vi "FGV_MCA.vi"(8 "Error In":errorcluster, 9 "TAC Settings":cluster{"Full Scale (ns)":dbl, "# bins":i32}={"Full Scale (ns)"=1000.0, "# bins"=1000} {"# bins" min=1 max=65535 step=1; "Full Scale (ns)" format="%0.2f"}, 10 "MCA Action":T1) -> (0 "error out":errorcluster, 1 "Delta Time (s)":dbl, 2 "Total Time (s)":dbl, 3 "Coincidence Signal":cluster{"Axis":dbl[], i32[]}(graph), 5 "Paused":bool)   [LabVIEW 2014]
doc: "Functional Global Variable or Action Engine implementation of a Multi-Channel Analyser that uses a DAQcard's analog input triggered by a logic pulse received on digital trigger input.\n\nBy default the analog input range is set from 0 V to 10 V full scale. The read trigger digital pulse arrives on PFI14 (pin 41), and the analog differential read on AI0+ and AI0-.\n\nTested on both M and X series DAQcards."
uses:
  Typedef_MCAControl.ctl
  <vilib>/DAQmx/read.llb/DAQmx Read (Analog 1D DBL 1Chan NSamp).vi
  <vilib>/DAQmx/create/channels.llb/DAQmx Create Channel (AI-Voltage-Basic).vi
  <vilib>/DAQmx/configure/timing.llb/DAQmx Timing (Sample Clock).vi
  <vilib>/DAQmx/miscellaneous.llb/DAQmx Fill In Error Info.vi
  <vilib>/Analysis/NI_AALPro.lvlib
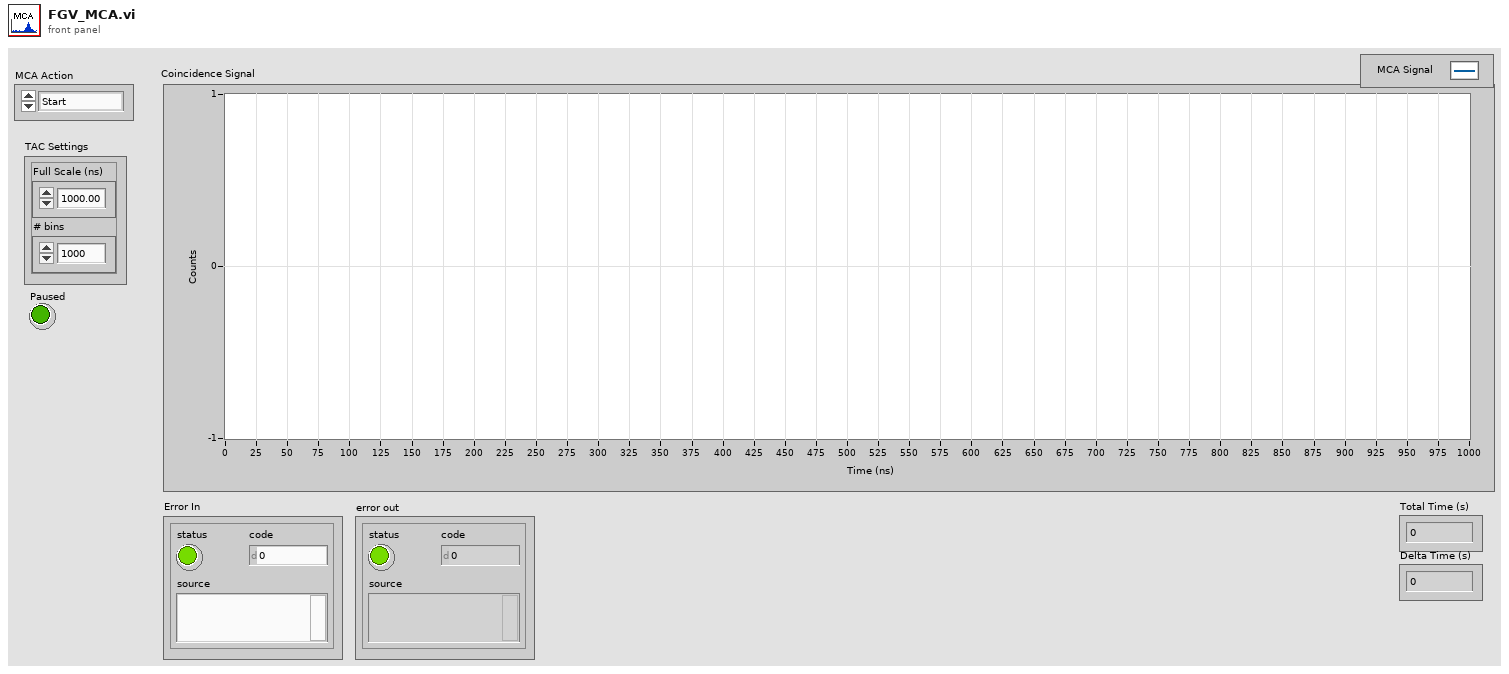
[diagram p1: front panel]
types:
  T1 = typedef "Typedef_MCAControl.ctl" = enum16{"Start", "Check", "Pause", "Unpause", "Update Settings", "Reset", "Stop"}
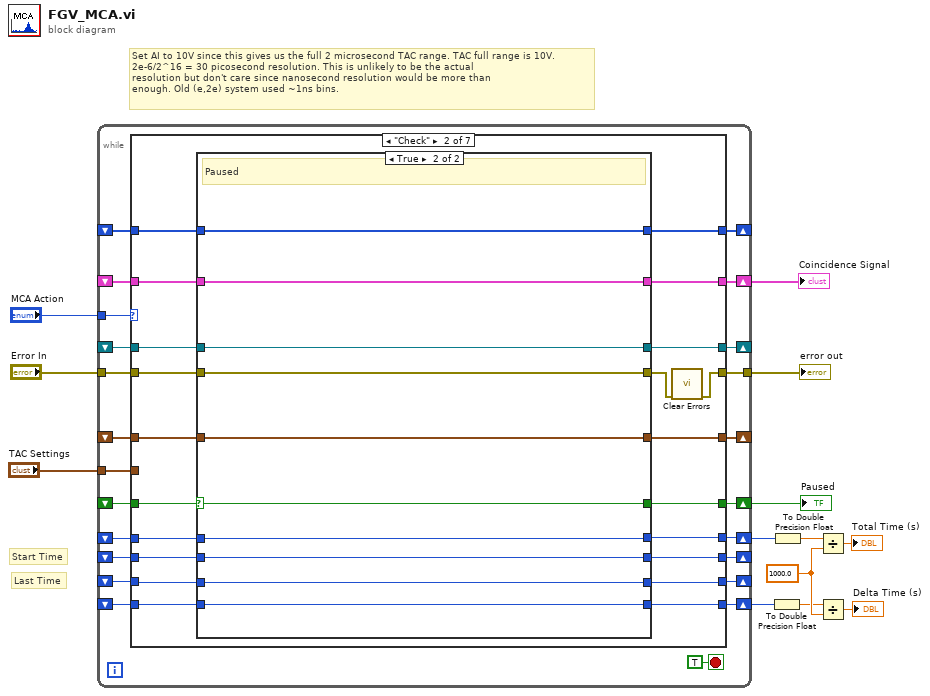
[diagram p0: block diagram]
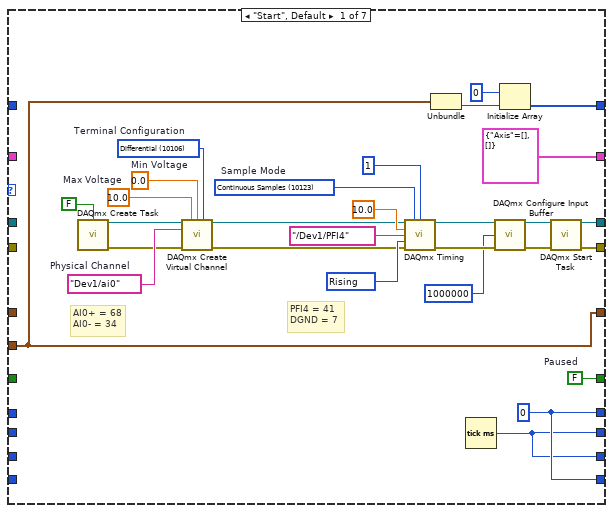
[diagram p2: hidden frame]
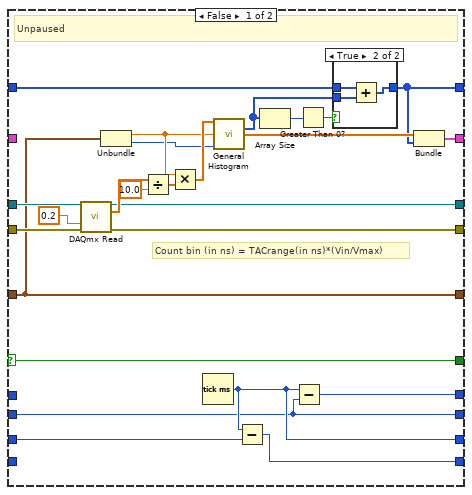
[diagram p3: hidden frame]
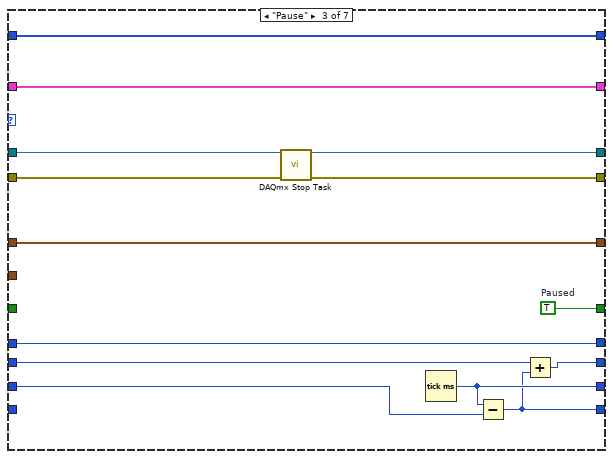
[diagram p5: hidden frame]
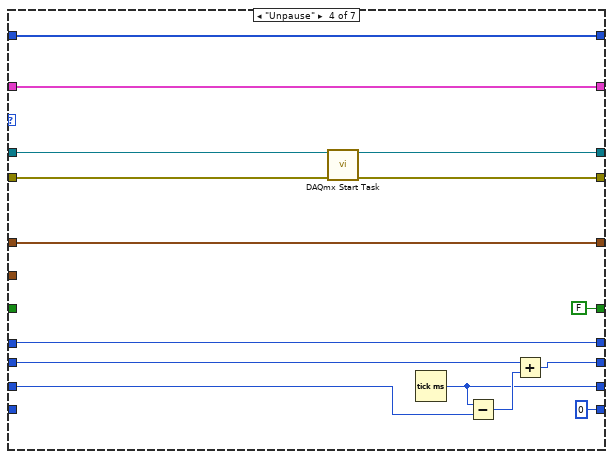
[diagram p6: hidden frame]
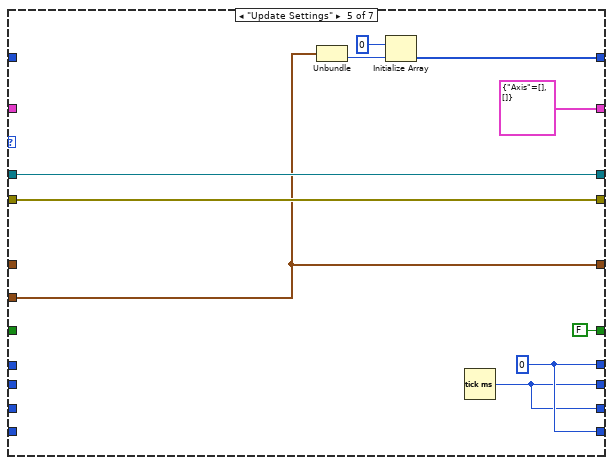
[diagram p7: hidden frame]
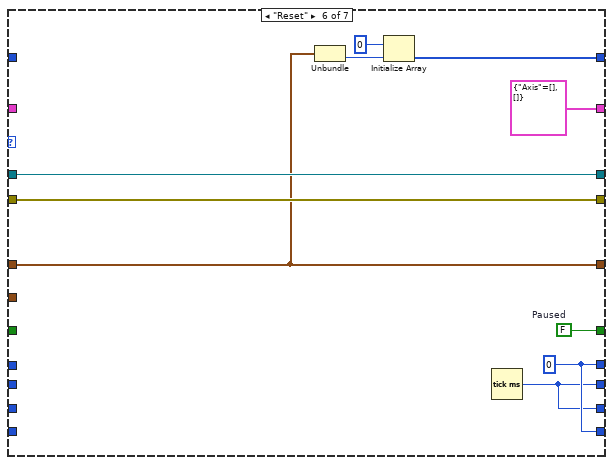
[diagram p8: hidden frame]
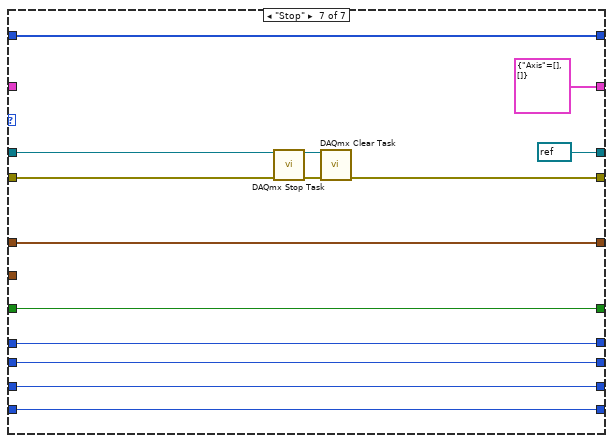
[diagram p9: hidden frame]
diagram:
  w6 = 1000.0 ("x")
  # "Last Time"
  # "Start Time"
  # "Set AI to 10V since this gives us the full 2 microsecond TAC range. TAC full range is 10V.\n2e-6/2^16 = 30 picosecond resolution. This is unlikely to be the actual\nresolution but don't care since nanosecond resolution would be more than\nenough. Old (e,2e) system used ~1ns bins."
  n1 = while {
    tunnel: "MCA Action" -> [w33]
    shift-right: [w35] -> _
    shift-left: _ -> [w34]
    shift-right: [w30] -> _
    shift-left: _ -> [w31]
    shift-right: [w27] -> _
    shift-left: _ -> [w29]
    tunnel: "TAC Settings" -> [w26]
    tunnel: "Error In" -> [w25]
    tunnel: [w36] -> w13
    shift-right: [w28] -> w11
    shift-left: _ -> [w24]
    shift-right: [w23] -> w8
    shift-left: _ -> [w22]
    shift-right: [w20] -> w1
    shift-left: _ -> [w17]
    shift-right: [w21] -> _
    shift-left: _ -> [w16]
    shift-right: [w18] -> _
    shift-left: _ -> [w15]
    shift-right: [w19] -> w2
    shift-left: _ -> [w14]
    stop <- TRUE stop-if-true
    n2 = case shown="\"Check\"" w33 {
      tunnel: [w57 w66 w135 w140 w164 w174 w185] -> w36
      tunnel: [w56 w84 w136 w142 w163 w173 refnum<k21> refnum ("task out")] -> w35
      tunnel: w34 -> [_ w85 w137 w143 w163 w173 w184]
      tunnel: w25 -> [_ w86 w138 w141 w164 w174 w186]
      tunnel: w31 -> [_ w83 w133 w154 _ _ w182]
      tunnel: [w51 w82 w133 w154 w157 w170 w182] -> w30
      tunnel: w29 -> [_ w80 w139 w152 _ w165 w180]
      tunnel: [cluster{"Axis":dbl[], i32[]} {"Axis"=[], []} w81 w134 w153 cluster{"Axis":dbl[], i32[]} {"Axis"=[], []} cluster{"Axis":dbl[], i32[]} {"Axis"=[], []} cluster{"Axis":dbl[], i32[]} {"Axis"=[], []}] -> w28
      tunnel: [w49 w78 w139 w152 w156 w165 w180] -> w27
      tunnel: w26 -> [w49 _ _ _ w156 _ _]
      tunnel: w24 -> [_ w79 w134 w153 _ _ _]
      tunnel: [w39 w76 w132 FALSE ("Paused") FALSE ("Paused") w168 w179] -> w23
      tunnel: w22 -> [_ w77 _ _ _ _ w179]
      tunnel: [w37 w73 w130 w148 w160 w166 w177] -> w21
      tunnel: [w38 w72 w131 w147 w161 w167 w178] -> w20
      tunnel: [w38 w75 w126 u32 0 w161 w167 w175] -> w19
      tunnel: [w37 w74 w127 w149 w160 w166 w176] -> w18
      tunnel: w17 -> [_ w69 w131 w147 _ _ w178]
      tunnel: w16 -> [_ w71 w129 w146 _ _ w177]
      tunnel: w15 -> [_ w70 w128 w145 _ _ w176]
      tunnel: w14 -> [_ w68 _ _ _ _ w175]
      frame "Start", Default {
        w38 = u32 0
        w39 = FALSE  # Paused
        w58 = tag "Dev1/ai0"  # Physical Channel
        w63 = 10.0  # Max Voltage
        w62 = 0.0  # Min Voltage
        w59 = 10106 items=["default"=-1, "RSE"=10083, "NRSE"=10078, "Differential"=10106, "Pseudodifferential"=12529]  # Terminal Configuration
        w65 = 10280 items=["Rising"=10280, "Falling"=10171] ("active edge")
        w53 = 10123 items=["Finite Samples"=10178, "Continuous Samples"=10123, "Hardware Timed Single Point"=12522]  # Sample Mode
        # "AI0+ = 68\nAI0- = 34"
        # "PFI4 = 41\nDGND = 7"
        n3 = call <vilib>:"DAQmx Create Task.vi"("auto cleanup"=FALSE) -> ("task out"=w47:refnum<k21>, "error out"=w46:errorcluster)  [unwired: 13 in]
        n4 = call-poly <vilib>:"DAQmx Create Virtual Channel.vi"("task in"=w47, "maximum value"=w63, "minimum value"=w62, "input terminal configuration"=w59, "physical channels"=w58, "error in"=w46) -> ("task out"=w55:refnum<k21>, "error out"=w54:errorcluster)  [unwired: 8 in]
        n5 = call-poly <vilib>:"DAQmx Timing.vi"("task/channels in"=w55, "sample mode"=w53, "samples per channel"=1 ("Number of Samples"), "rate"=10.0 ("Sample Rate"), "source"=tag "/Dev1/PFI4" ("Sample Clock Source"), "active edge"=w65, "error in"=w54) -> ("task out"=w43:refnum<k21>, "error out"=w42:errorcluster)  [unwired: 7 in]
        n6 = Unbundle(w49) -> ("# bins"=w40:i32)  [unwired: 1 out]
        n7 = Tick Count (ms)() -> (millisecond timer value=w37:u32)
        n8 = call <vilib>:"DAQmx Configure Input Buffer.vi"("task/channels in"=w43, "buffer size (in samples per channel)"=u32 1000000, "error in"=w42) -> ("task out"=w44:refnum<k21>, "error out"=w45:errorcluster)  [unwired: 11 in]
        n9 = Initialize Array(0 ("element"), w40) -> (w51:i32[])
        n10 = call <vilib>:"DAQmx Start Task.vi"("task/channels in"=w44, "error in"=w45) -> ("task out"=w56:refnum<k21>, "error out"=w57:errorcluster)  [unwired: 12 in]
      }
      frame "Check" {
        n11 = case shown="True" w77 {
          selector: w77 -> [w92 w120]
          tunnel: w86 -> [w102 w122]
          tunnel: w85 -> [w101 w123]
          tunnel: [w100 w122] -> w67
          tunnel: [w99 w123] -> w84
          tunnel: w83 -> [w98 w125]
          tunnel: [w97 w125] -> w82
          tunnel: [w96 w124] -> w81
          tunnel: w80 -> [w93 w121]
          tunnel: w79 -> [_ w124]
          tunnel: [w93 w121] -> w78
          tunnel: [w92 w120] -> w76
          tunnel: [w91 w116] -> w75
          tunnel: [w90 w117] -> w74
          tunnel: [w88 w118] -> w73
          tunnel: [w89 w119] -> w72
          tunnel: w71 -> [w88 w118]
          tunnel: w70 -> [w87 w117]
          tunnel: w69 -> [_ w119]
          tunnel: w68 -> [_ w116]
          frame False {
            # "Count bin (in ns) = TACrange(in ns)*(Vin/Vmax)"
            # "Unpaused"
            n12 = call-poly <vilib>:"DAQmx Read.vi"("task/channels in"=w101, "timeout"=0.2, "error in"=w102) -> ("task out"=w99:refnum<k21>, "data"=w106:dbl[], "error out"=w100:errorcluster)  [unwired: 10 in]
            n13 = Unbundle(w93) -> ("Full Scale (ns)"=w95:dbl, "# bins"=w94:i32)
            n14 = Divide(x=w106, y=10.0 ("Waveform")) -> (x/y=w104:dbl[])
            n15 = Multiply(x=w95, y=w104) -> (x*y=w103:dbl[])
            n16 = Tick Count (ms)() -> (millisecond timer value=w90:u32)
            n17 = call <vilib>:"General Histogram.vi"("X"=w103, "max"=w95, "# bins"=w94) -> ("Histogram"=w107:i32[], "Axis"=w110:dbl[])  [unwired: 3 in, 8 out]
            n18 = Subtract(x=w90, y=w87) -> (x-y=w91:u32)
            n19 = Array Size(array=w107) -> (size(s)=w109:i32)
            n20 = Subtract(x=w90, y=w88) -> (x-y=w89:u32)
            n21 = Greater Than 0?(x=w109) -> (x > 0?=w108:bool)
            n22 = case shown="True" w108 {
              tunnel: w98 -> [w112 w115]
              tunnel: w107 -> [_ w114]
              tunnel: [w112 w113] -> w97
              frame False {
              }
              frame True {
                n23 = Add(x=w115, y=w114) -> (x+y=w113:i32[])
              }
            }
            n24 = Bundle("Axis"=w110, w97) -> (w96:cluster{"Axis":dbl[], i32[]})  [unwired: 1 out]
          }
          frame True {
            # "Paused"
          }
        }
        n25 = call <vilib>:"Clear Errors.vi"("error in (no error)"=w67) -> ("error out"=w66:errorcluster)  [unwired: 5 in, 1 out]
      }
      frame "Pause" {
        w132 = TRUE  # Paused
        n26 = call <vilib>:"DAQmx Stop Task.vi"("task/channels in"=w137, "error in"=w138) -> ("task out"=w136:refnum<k21>, "error out"=w135:errorcluster)  [unwired: 12 in]
        n27 = Tick Count (ms)() -> (millisecond timer value=w127:u32)
        n28 = Subtract(x=w127, y=w128) -> (x-y=w126:u32)
        n29 = Add(x=w129, y=w126) -> (x+y=w130:u32)
      }
      frame "Unpause" {
        n30 = call <vilib>:"DAQmx Start Task.vi"("task/channels in"=w143, "error in"=w141) -> ("task out"=w142:refnum<k21>, "error out"=w140:errorcluster)  [unwired: 12 in]
        n31 = Tick Count (ms)() -> (millisecond timer value=w149:u32)
        n32 = Subtract(x=w149, y=w145) -> (x-y=w150:u32)
        n33 = Add(x=w146, y=w150) -> (x+y=w148:u32)
      }
      frame "Update Settings" {
        w161 = u32 0
        n34 = Unbundle(w156) -> ("# bins"=w158:i32)  [unwired: 1 out]
        n35 = Initialize Array(0 ("element"), w158) -> (w157:i32[])
        n36 = Tick Count (ms)() -> (millisecond timer value=w160:u32)
      }
      frame "Reset" {
        w167 = u32 0
        w168 = FALSE  # Paused
        n37 = Unbundle(w165) -> ("# bins"=w171:i32)  [unwired: 1 out]
        n38 = Initialize Array(0 ("element"), w171) -> (w170:i32[])
        n39 = Tick Count (ms)() -> (millisecond timer value=w166:u32)
      }
      frame "Stop" {
        n40 = call <vilib>:"DAQmx Stop Task.vi"("task/channels in"=w184, "error in"=w186) -> ("task out"=w187:refnum<k21>, "error out"=w188:errorcluster)  [unwired: 12 in]
        n41 = call <vilib>:"DAQmx Clear Task.vi"("task in"=w187, "error in"=w188) -> ("error out"=w185:errorcluster)  [unwired: 13 in]
      }
    }
  }
  "error out" <- w13
  "Coincidence Signal" <- w11
  "Paused" <- w8
  n42 = To Double Precision Float(number=w2) -> (double precision float=w4:dbl)
  n43 = To Double Precision Float(number=w1) -> (double precision float=w3:dbl)
  n44 = Divide(x=w3, y=w6) -> (x/y=→"Total Time (s)":dbl)
  n45 = Divide(x=w4, y=w6) -> (x/y=→"Delta Time (s)":dbl)
